vi "Sidecar Controller.vi"(8 "error in":errorcluster) -> ()   [LabVIEW 2017]
doc: "This VI executes continuously carrying out the current operation and responding to updates or new operations. It will often contain the timing or control code that is difficult to place directly in TeleOp. This VI generally opens all sensors and motors and isolates the rest of the robot code from knowing how the operations are carried out."
uses:
  <vilib>/Rock Robotics/WPI/Framework/Completion Status.ctl
  Sidecar Setpoints.ctl
  Sidecar Operations.ctl
  <vilib>/Rock Robotics/SystemInterfaces/DIO/FPGA_DIOPWMChannel.ctl
  <vilib>/Rock Robotics/Network Tables/NT Write Boolean.vi
panel:
  out "Servo Position":u16(graph)
  out "Servo Position":i32
  out "error out":errorcluster
  in  "Interactive Values":T1
  out "Current\nCmd":string
  in  "Buttons":cluster{"Execute Cmd":bool, "Abort Cmd":bool}
  out "Command Timing":cluster{"Start Time (ms)":u32, "Iterations":i32}
  out "Status":T3
  # "Tip: It may be helpful to observe inputs and sensor values.\nYou may also want to display tuning or debugging controls."
  # "Interactive Command: You may fill in the settings for a command\nand schedule it with the Execute button. You can observe and abort\nany command while fine tuning the code for the controller."
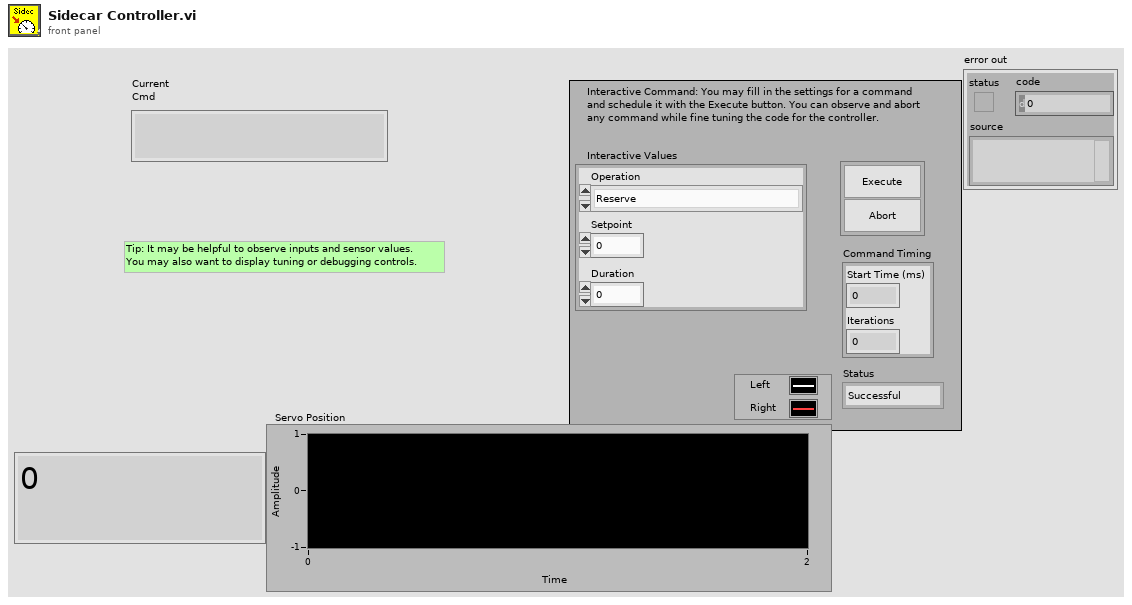
[diagram p1: front panel]
types:
  T1 = typedef "Sidecar Setpoints.ctl" = cluster{"Operation":T2, "Setpoint":dbl, "Duration":dbl}
  T2 = typedef "Sidecar Operations.ctl" = enum16{"Reserve", "Read Current", "Immediate", "Move Backward", "Move Forward"}
  T3 = typedef "Completion Status.ctl" = enum16{"Successful", "Aborted", "Incomplete"}
  T4 = typedef "FPGA_DIOPWMChannel.ctl" = enum8{"PWM 0", "PWM 1", "PWM 2", "PWM 3", "PWM 4", "PWM 5", "PWM 6", "PWM 7", "PWM 8", "PWM 9", "PWM MXP 0", "PWM MXP 1", "PWM MXP 2", "PWM MXP 3", "PWM MXP 4", "PWM MXP 5", "PWM MXP 6", "PWM MXP 7", "PWM MXP 8", "PWM MXP 9", "Invalid"}
  T5 = typedef "WPI_ServoDeviceRef.ctl" = cluster{"DeviceStatus":errorcluster, "PWM Channel":T4, "DeadBand":T6}
  T6 = typedef "WPI_PWMDeadband.ctl" = cluster{"Name":string, "maxPositivePwm":i32, "minPositivePwm":i32, "centerPwm":i32, "maxNegativePwm":i32, "minNegativePwm":i32, "angularRange":u16}
  T7 = typedef "Command Status Info.ctl" = cluster{"Name":string, "Status":T3, "notifier out":T8}
  T8 = typedef "Completion Notifier.ctl" = refnum<notifier>
  T9 = cluster{"Current Command":T1, "Command Timing":cluster{"Start Time (ms)":u32, "Iterations":i32}, "Command Arguments":cluster{"Command Info":T7, "Description":string, "Default Command":T1, "queue out":refnum<queue>, "Subsystem Name":string}}
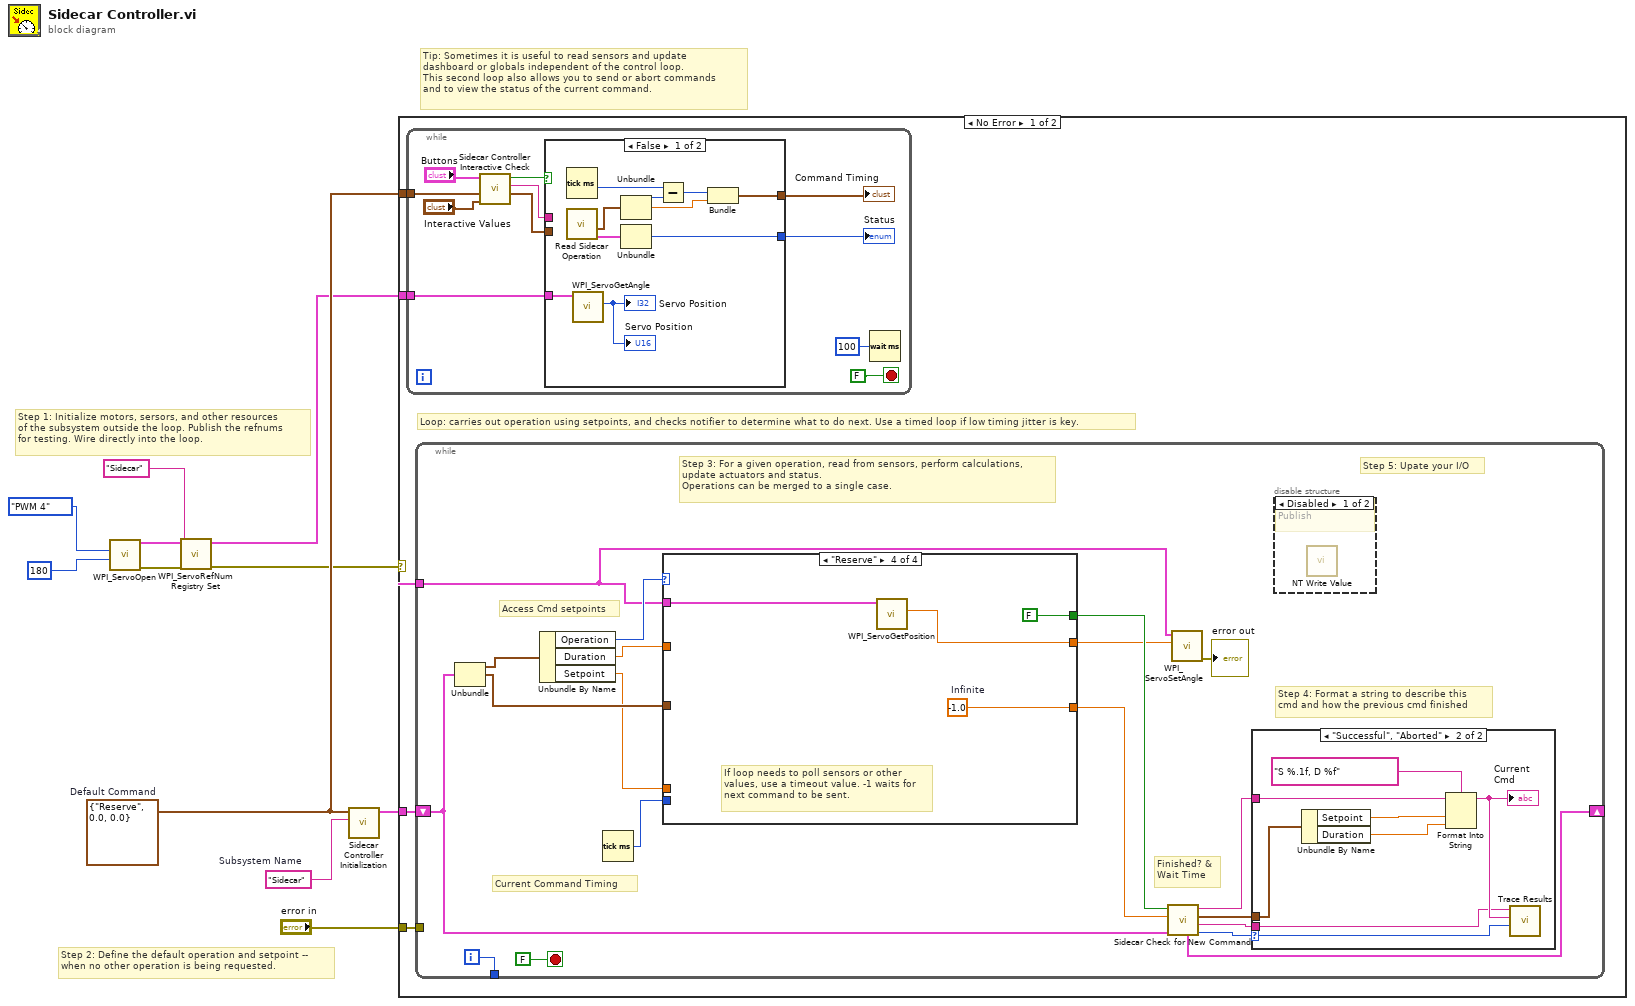
[diagram p0: block diagram]
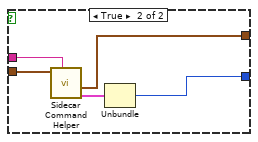
[diagram p2: hidden frame]
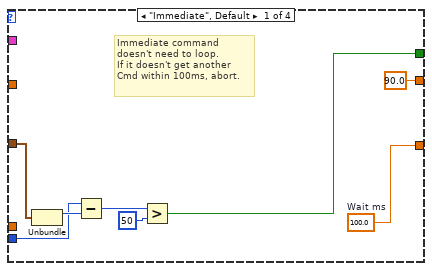
[diagram p5: hidden frame]
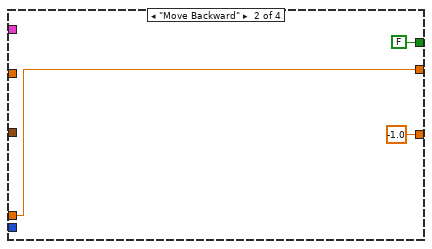
[diagram p6: hidden frame]
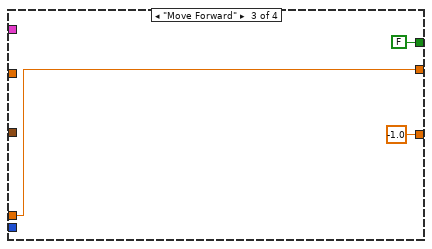
[diagram p7: hidden frame]
diagram:
  w8 = T1 {"Operation"=enum."Reserve", "Setpoint"=0.0, "Duration"=0.0}  # Default Command
  w9 = "Sidecar"  # Subsystem Name
  # "Tip: Sometimes it is useful to read sensors and update\ndashboard or globals independent of the control loop.\nThis second loop also allows you to send or abort commands\nand to view the status of the current command."
  # "Step 2: Define the default operation and setpoint --\nwhen no other operation is being requested."
  # "Step 1: Initialize motors, sersors, and other resources\nof the subsystem outside the loop. Publish the refnums\nfor testing. Wire directly into the loop."
  n1 = call <vilib>:"WPI_ServoOpen.vi"("Angular Range"=u16 180, "PWM Channel"=FPGA_DIOPWMChannel."PWM 4") -> ("error out"=w2:errorcluster, "ServoDeviceRef"=w5:T5)  [unwired: 8 in]
  n2 = call <vilib>:"WPI_ServoRefNum Registry Set.vi"("error in (no error)"=w2, "refnum name"="Sidecar", "ServoDeviceRef"=w5) -> ("error out"=w1:errorcluster, "ServoDeviceRef"=w3:T5)  [unwired: 7 in]
  n3 = call "Sidecar Controller Initialization.vi"("Subsystem Name"=w9, "Default Command"=w8) -> ("Current Command"=w10:T9)  [unwired: 9 in]
  n4 = case shown="No Error" w1 {
    tunnel: "error in" -> [w15 _]
    tunnel: w10 -> [w14 _]
    tunnel: w8 -> [w13 _]
    tunnel: w3 -> [w12 _]
    frame No Error {
      # "Loop: carries out operation using setpoints, and checks notifier to determine what to do next. Use a timed loop if low timing jitter is key."
      n5 = while {
        tunnel: w13 -> [w23]
        tunnel: w12 -> [w16]
        stop <- FALSE stop-if-true
        n6 = call "Sidecar Controller Interactive Check.vi"("Interactive Command in"="Interactive Values", "Default Command"=w23, "Buttons"="Buttons") -> ("Interactive Command out"=w20:T1, "Trace String"=w21:string, "Schedule"=w22:bool)  [unwired: 6 in]
        n7 = case shown="False" w22 {
          tunnel: [w36 w41] -> w19
          tunnel: w20 -> [_ w39]
          tunnel: [w32 w37] -> w18
          tunnel: w21 -> [_ w40]
          tunnel: w16 -> [w28 _]
          frame False {
            n8 = Tick Count (ms)() -> (millisecond timer value=w31:u32)
            n9 = call "Read Sidecar Operation.vi"() -> ("Command Info"=w29:T7, "SubSystem Data"=w30:T1)  [unwired: 9 in, 1 out]
            n10 = call <vilib>:"WPI_ServoGetAngle.vi"("ServoDeviceRef"=w28) -> ("Angle"=→"Servo Position" →"Servo Position":u16)  [unwired: 7 in, 2 out]
            n11 = Unbundle(w30) -> ("Operation"=w35:T2, "Setpoint"=w33:dbl)  [unwired: 1 out]
            n12 = Unbundle(w29) -> ("Status"=w36:T3)  [unwired: 2 out]
            n13 = Subtract(x=w31, y=w35) -> (x-y=w34:u32)
            n14 = Bundle(w34, "Setpoint"=w33) -> (w32:cluster{u32, "Setpoint":dbl})  [unwired: 1 in]
          }
          frame True {
            n15 = call "Sidecar Command Helper.vi"("Description"=w40, "SubSystem Data"=w39) -> ("Command Info Out"=w38:T7, "Command Timing"=w37:cluster{"Start Time (ms)":u32, "Iterations":i32})  [unwired: 7 in, 1 out]
            n16 = Unbundle(w38) -> ("Status"=w41:T3)  [unwired: 2 out]
          }
        }
        "Status" <- w19
        "Command Timing" <- w18
        n17 = Wait (ms)(milliseconds to wait=u32 100) -> ()  [unwired: 1 out]
      }
      n18 = while {
        shift-right: [w52] -> _
        shift-left: w14 -> [w45]
        tunnel: [w59] -> _
        tunnel: w15 -> [_]
        tunnel: w12 -> [w44]
        i -> [w59]
        stop <- FALSE stop-if-true
        # "Step 5: Upate your I/O"
        # "Step 4: Format a string to describe this\ncmd and how the previous cmd finished"
        # "Current Command Timing"
        # "Access Cmd setpoints"
        # "Finished? &\nWait Time"
        # "Step 3: For a given operation, read from sensors, perform calculations,\nupdate actuators and status.\nOperations can be merged to a single case."
        n19 = Unbundle(w45) -> ("Current Command"=w58:T1, "Command Timing"=w54:cluster{"Start Time (ms)":u32, "Iterations":i32})  [unwired: 1 out]
        n20 = Unbundle By Name(w58) -> ("Operation"=w57:T2, "Duration"=w56:dbl, "Setpoint"=w53:dbl)
        n21 = Tick Count (ms)() -> (millisecond timer value=w55:u32)
        n22 = case shown="\"Reserve\"" w57 {
          tunnel: [w76 -1.0 ("Infinite") -1.0 ("Infinite") w86] -> w50
          tunnel: [w70 FALSE ("ignore previous (F)") FALSE ("ignore previous (F)") FALSE ("ignore previous (F)")] -> w51
          tunnel: w54 -> [w72 _ _ _]
          tunnel: w56 -> [_ _ _ _]
          tunnel: w55 -> [w71 _ _ _]
          tunnel: w53 -> [_ w79 w81 _]
          tunnel: w44 -> [_ _ _ w84]
          tunnel: [90.0 ("Position") w79 w81 w83] -> w43
          frame "Immediate", Default {
            w76 = 100.0  # Wait ms
            # "Immediate command\ndoesn't need to loop.\nIf it doesn't get another\nCmd within 100ms, abort."
            n23 = Unbundle(w72) -> ("Start Time (ms)"=w75:u32)  [unwired: 1 out]
            n24 = Subtract(x=w71, y=w75) -> (x-y=w74:u32)
            n25 = Greater?(x=w74, y=u8 50 ("Left Motor")) -> (0:w70:bool)
          }
          frame "Move Backward" {
          }
          frame "Move Forward" {
          }
          frame "Reserve" {
            w86 = -1.0  # Infinite
            # "If loop needs to poll sensors or other\nvalues, use a timeout value. -1 waits for\nnext command to be sent."
            n26 = call <vilib>:"WPI_ServoGetPosition.vi"("ServoDeviceRef"=w84) -> ("Position"=w83:dbl)  [unwired: 8 in, 2 out]
          }
        }
        n27 = call "Sidecar Check for New Command.vi"("Current Command"=w45, "Wait time (ms)"=w50, "Finished?"=w51) -> ("Completion"=w46:T3, "Subsystem Name"=w47:string, "Current Command"=w48:T1, "Initial Trace String"=w49:string, "NextCommand"=w52:T9)  [unwired: 4 in]
        n28 = call <vilib>:"WPI_ServoSetAngle.vi"("Angle"=w43, "ServoDeviceRef"=w44) -> ("error out"=→"error out":errorcluster)  [unwired: 8 in, 1 out]
        n29 = case shown="\"Successful\", \"Aborted\"" w46 {
          selector: w46 -> [_ w68]
          tunnel: w49 -> [_ w64]
          tunnel: w48 -> [_ w65]
          tunnel: w47 -> [_ w61]
          frame "Incomplete", Default {
            # "Continuing current command"
          }
          frame "Successful", "Aborted" {
            # "Report and setup for next command"
            n30 = Unbundle By Name(w65) -> ("Setpoint"=w67:dbl, "Duration"=w62:dbl)
            n31 = Format Into String(format string="S %.1f, D %f", initial string=w64, w67, w62) -> (resulting string=w63:string)  [unwired: 1 in, 1 out]
            "Current\nCmd" <- w63
            n32 = call <vilib>:"Trace Results.vi"("Status of previous command"=w68, "Description"=w63, "Subsystem"=w61) -> ()  [unwired: 9 in]
          }
        }
        n33 = disable-structure shown="Disabled" {
          frame Disabled {
            # "Publish"
            n34 = call-poly <vilib>:"NT Write Value.vi"() -> ()  [unwired: 11 in, 1 out]
          }
          frame Enabled {
          }
        }
      }
    }
    frame Error {
    }
  }
